vi "ReferenceMove.vi"(0 "object in":refnum<class "CetoniPump.lvclass">, 2 "index":i32, 5 "error in (no error)":errorcluster) -> (14 "object out":refnum<class "CetoniPump.lvclass">, 19 "error out":errorcluster)   [LabVIEW 2021, in "CetoniPump.lvclass"]
uses:
  CetoniPump.lvclass
  CetoniPump.lvclass/CetoniPump.ctl
  Users/olaja/AppData/Local/CETONI_SDK/lib/labview/labbCAN_Pump_API/labbCAN_Pump_API.lvlib
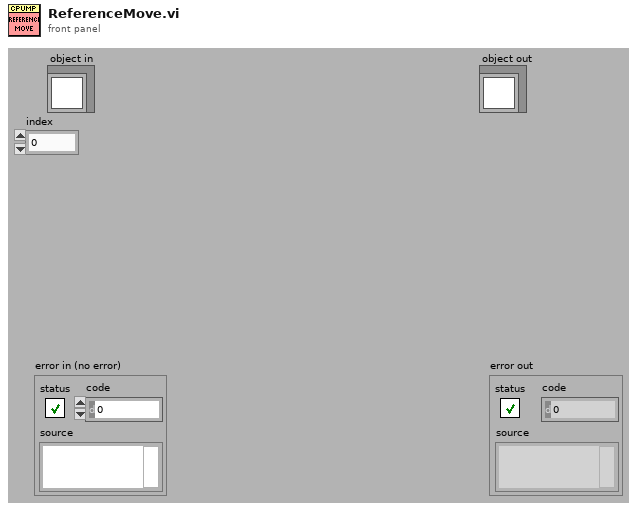
[diagram p1: front panel]
types:
  T1 = cluster{"Pump Handle":i64, "Pump Name":string, "Maximum Volume":dbl, "Maximum Flow Rate":dbl, "Flow Rate":dbl, "Fill Level":dbl}[]
  T2 = cluster{"Pump Handle":i64, "Pump Name":string, "Maximum Volume":dbl, "Maximum Flow Rate":dbl, "Flow Rate":dbl, "Fill Level":dbl}
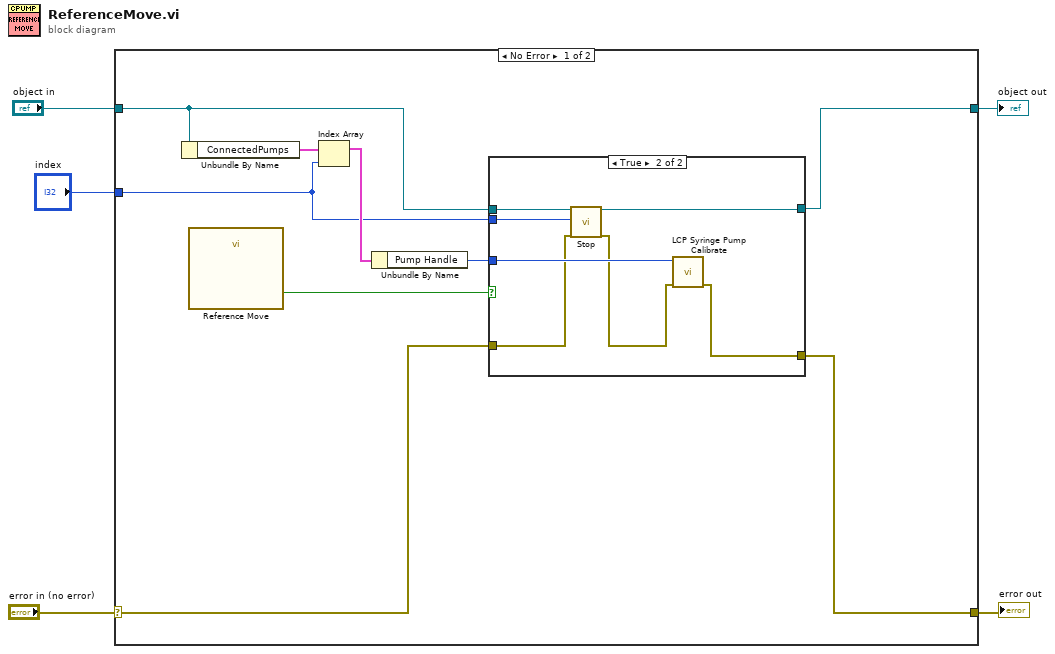
[diagram p0: block diagram]
diagram:
  n1 = case shown="No Error" "error in (no error)" {
    selector: "error in (no error)" -> [w13 w25]
    tunnel: [w12 w25] -> w4
    tunnel: [w10 w24] -> w2
    tunnel: "object in" -> [w9 w24]
    tunnel: "index" -> [w7 _]
    frame No Error {
      n2 = Unbundle By Name(w9) -> ("ConnectedPumps"=w14:T1)
      n3 = call "Reference Move"() -> ("OK"=w11:bool)  [unwired: 18 in, 1 out]
      n4 = Index Array(array=w14, index=w7) -> (element=w8:T2)
      n5 = Unbundle By Name(w8) -> ("Pump Handle"=w6:i64)
      n6 = case shown="True" w11 {
        tunnel: w6 -> [_ w23]
        tunnel: w13 -> [w16 w19]
        tunnel: [w16 w22] -> w12
        tunnel: w9 -> [w15 w21]
        tunnel: [w15 w18] -> w10
        tunnel: w7 -> [_ w17]
        frame False {
        }
        frame True {
          n7 = call-dynamic "Stop.vi"("object in"=w21, "index"=w17, "error in (no error)"=w19) -> ("object out"=w18:refnum<class "CetoniPump.lvclass">, "error out"=w20:errorcluster)  [unwired: 15 in]
          n8 = call "LCP Syringe Pump Calibrate.vi"("error in (no error)"=w20, "Pump Handle"=w23) -> ("error out"=w22:errorcluster)  [unwired: 9 in]
        }
      }
    }
    frame Error {
    }
  }
  "error out" <- w4
  "object out" <- w2
